vi "Test Data.vi"() -> ()   [LabVIEW 2023]
panel:
  out "?":cluster{dbl, dbl}[](array[cluster])
  out "Data Det 1":T1(array[cluster])
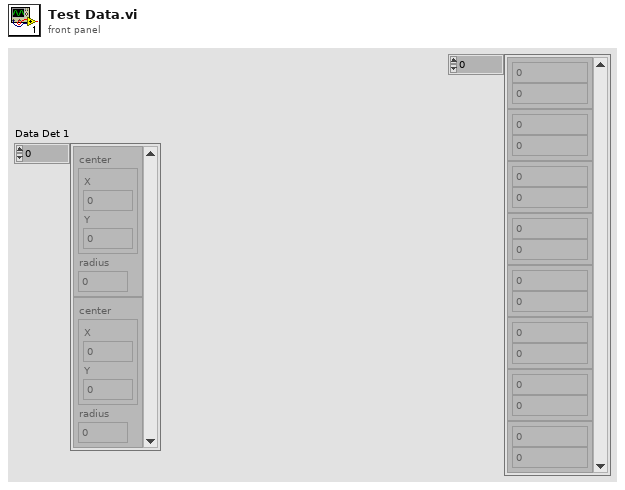
[diagram p1: front panel]
types:
  T1 = cluster{"center":cluster{"X":sgl, "Y":sgl}, "radius":sgl}[]
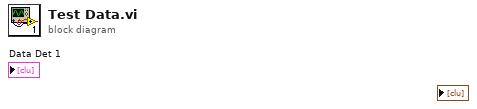
[diagram p0: block diagram]
diagram:
